vi "BotSpeakURAPI.vi"(2 "Translator":T1(array[cluster]), 3 "To Send":string) -> (0 "translated w \\n":string, 1 "translated":string)   [LabVIEW 2012]
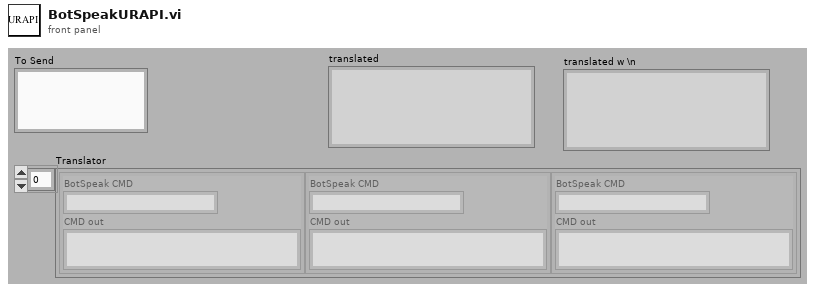
[diagram p1: front panel]
types:
  T1 = cluster{"BotSpeak CMD":string, "CMD out":string}[]
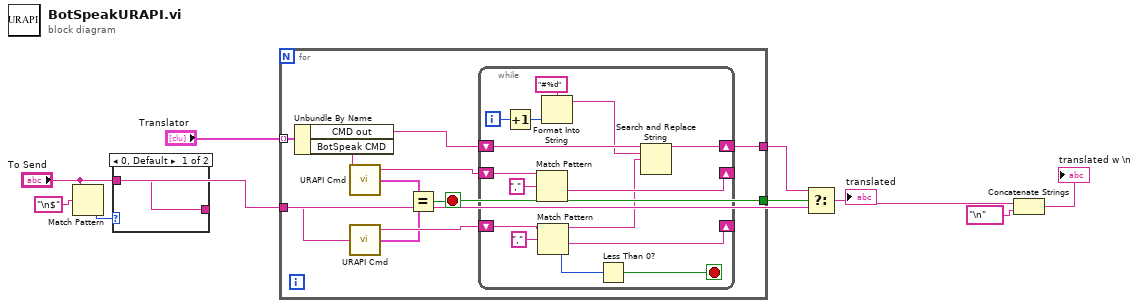
[diagram p0: block diagram]
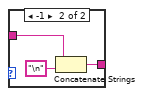
[diagram p2: hidden frame]
diagram:
  n1 = Match Pattern(string="To Send", regular expression="\n$" ("delimiter (Tab)")) -> (offset past match=w7:i32)  [unwired: 1 in, 3 out]
  n2 = case shown="0, Default" w7 {
    tunnel: [w10 w13] -> _
    tunnel: "To Send" -> [w10 w11]
    frame 0, Default {
    }
    frame -1 {
      n3 = Concatenate Strings(w11, "\n" ("string")) -> (w13:string)
    }
  }
  n4 = for {
    tunnel: "Translator" -> [w23] mode=indexing
    tunnel: "To Send" -> [w17]
    tunnel: [w20] -> w3
    tunnel: [w19] -> w4
    stop <- w19 stop-if-true
    n5 = Unbundle By Name(w23) -> ("CMD out"=w21:string, "BotSpeak CMD"=w18:string)
    n6 = call <userlib>:"URAPI Cmd.vi"("BotSpeak CMD"=w18) -> ("Command"=w15:cluster{"CMD":string, "# params":i32}, "Params"=w22:string)  [unwired: 1 in]
    n7 = call <userlib>:"URAPI Cmd.vi"("BotSpeak CMD"=w17) -> ("Command"=w14:cluster{"CMD":string, "# params":i32}, "Params"=w16:string)  [unwired: 1 in]
    n8 = Equal?(x=w15, y=w14) -> (x = y?=w19:bool)
    n9 = while {
      shift-right: [w34] -> _
      shift-left: w22 -> [w37]
      shift-right: [w33] -> _
      shift-left: w16 -> [w35]
      shift-right: [w30] -> w20
      shift-left: w21 -> [w31]
      i -> [w29]
      stop <- w24 stop-if-true
      n10 = Increment(x=w29) -> (x+1=w26:i32)
      n11 = Match Pattern(string=w37, regular expression=",") -> (after substring=w34:string)  [unwired: 1 in, 3 out]
      n12 = Match Pattern(string=w35, regular expression=",") -> (before substring=w32:string, after substring=w33:string, offset past match=w25:i32)  [unwired: 1 in, 1 out]
      n13 = Format Into String(format string="#%d", w26) -> (resulting string=w27:string)  [unwired: 2 in, 1 out]
      n14 = Less Than 0?(x=w25) -> (x < 0?=w24:bool)
      n15 = Search and Replace String(input string=w31, search string=w27, replace string=w32) -> (result string=w30:string)  [unwired: 5 in, 3 out]
    }
  }
  n16 = Select(t=w3, s=w4, f="To Send") -> (s? t:f=w1:string)
  "translated" <- w1
  n17 = Concatenate Strings(w1, "\n" ("delimiter (Tab)")) -> (→"translated w \\n":string)
